vi "Create.vi"(7 "Size (-1, Unlimited)":i32, 8 "error in (no error)":errorcluster) -> (0 "error out":errorcluster, 3 "MessageQ out":refnum<class "MessageQ.lvclass">)   [LabVIEW 2020, in "Volatus.lvlib" / "MessageQ.lvclass"]
uses:
  MessageQ.lvclass
  MessageQ.lvclass/MessageQ.ctl
  Message.ctl
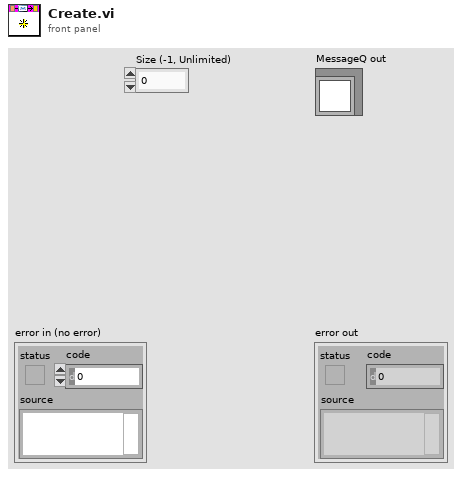
[diagram p1: front panel]
types:
  T1 = typedef "Volatus.lvlib/MessageQ.lvclass/Message.ctl" = cluster{"ID":string, "Data":variant}
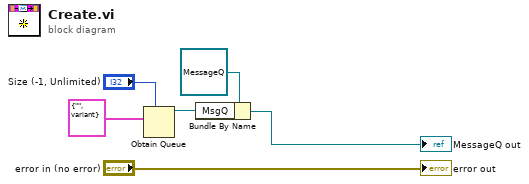
[diagram p0: block diagram]
diagram:
  n1 = Obtain Queue(max queue size (-1, unlimited)="Size (-1, Unlimited)", element data type=T1 {"ID"="", "Data"=variant} ("Message")) -> (queue out=w1:refnum<queue>)  [unwired: 3 in, 2 out]
  n2 = Bundle By Name(cluster=refnum<class "MessageQ.lvclass"> refnum ("MessageQ in"), "MsgQ"=w1) -> (→"MessageQ out":refnum<class "MessageQ.lvclass">)
  "error out" <- "error in (no error)"
